vi "sin_glob.vi"(11 "dx":dbl) -> (3 "sin(x)":dbl)   [LabVIEW 2022 SP3]
uses:
  x_var.vi
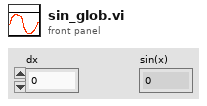
[diagram p1: front panel]
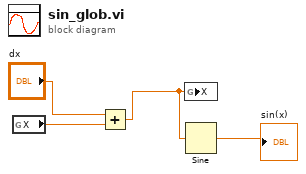
[diagram p0: block diagram]
diagram:
  n1 = global read "x_var.vi" "X"() -> (w3:dbl)
  n2 = Add(x="dx", y=w3) -> (x+y=w1:dbl)
  n3 = global write "x_var.vi" "X"(w1) -> ()
  n4 = Sine(x=w1) -> (sin(x)=→"sin(x)":dbl)
